vi "demo.vi"() -> ()   [LabVIEW 2009]
uses:
  <vilib>/Utility/miscctls.llb/LVPositionTypeDef.ctl
panel:
  in  "exit":bool
  in  "type":i8(ring) items=["甲", "乙", "丙", "丁"]
  in  "listbox":i32(listbox)
  # "演示列表框"
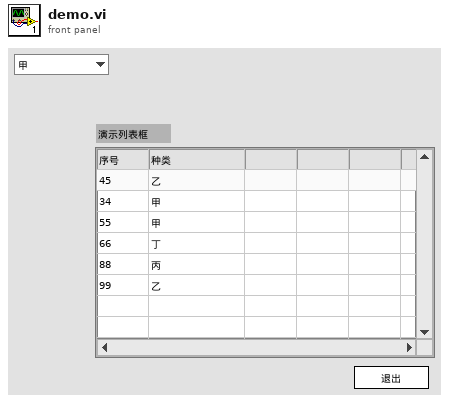
[diagram p1: front panel]
types:
  T1 = typedef "LVPositionTypeDef.ctl" = cluster{"Left":i32, "Top":i32}
  T2 = typedef "LVRowAndColumnTypeDef.ctl" = cluster{"Row":i32, "Column":i32}
  T3 = typedef "LVPoint32TypeDef.ctl" = cluster{"Horizontal":i32, "Vertical":i32}
  T4 = typedef "LVBoundsTypeDef.ctl" = cluster{"Width":u32, "Height":u32}
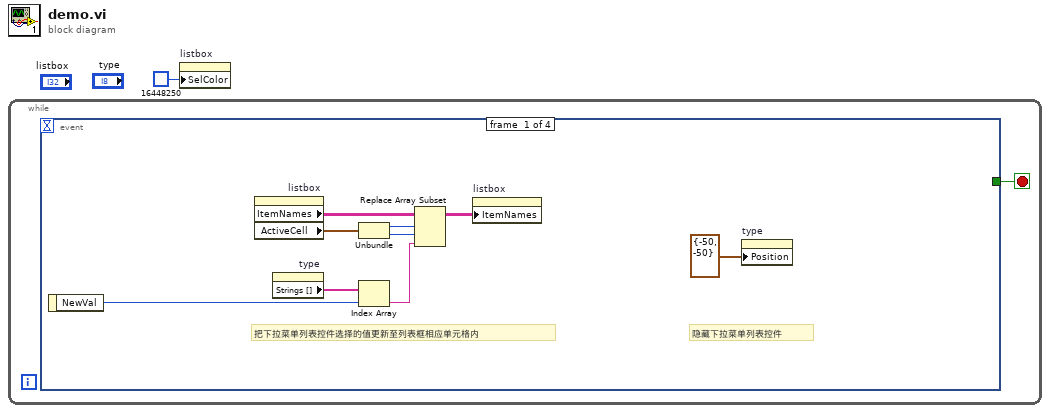
[diagram p0: block diagram]
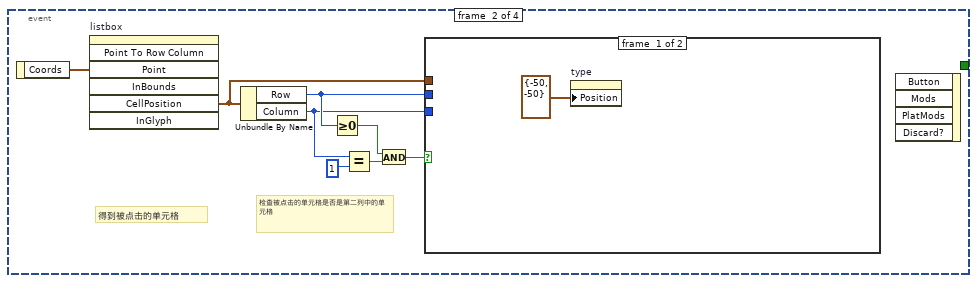
[diagram p2: hidden frame]
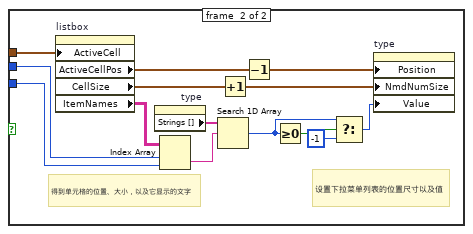
[diagram p3: hidden frame]
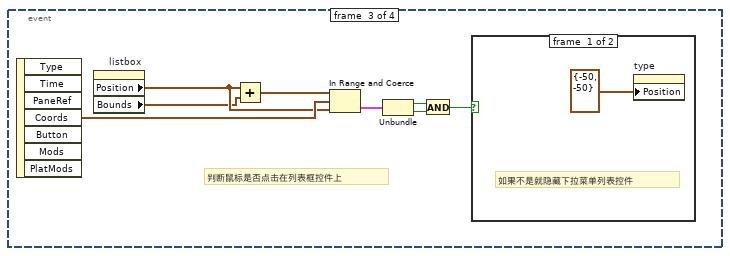
[diagram p4: hidden frame]
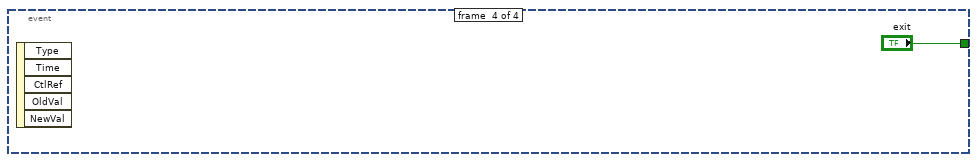
[diagram p6: hidden frame]
diagram:
  n1 = while {
    stop <- w2 stop-if-true
    n2 = event shown="[1] \"listbox\": Mouse Down?" {
      selector: _ -> [_ _ _ _]
      dyn-events: _ -> [_ _ _ _]
      timeout: _ -> [_ _ _ _]
      tunnel: [_ _ _ "exit"] -> w2
      event #0 {
        # "隐藏下拉菜单列表控件"
        # "把下拉菜单列表控件选择的值更新至列表框相应单元格内"
        n3 = event-data() -> ("NewVal"=w10:i8)  [unwired: 1 in]
        n4 = property on="listbox" class="MCListbox (strict)"() -> ("ItemNames"=w9:string[][], "ActiveCell"=w8:T2)  [unwired: 2 in, 2 out]
        n5 = property on="type" class="Ring (strict)"() -> ("Strings []"=w11:string[])  [unwired: 2 in, 2 out]
        n6 = Unbundle(w8) -> ("Row"=w7:i32, "Column"=w6:i32)
        n7 = Index Array(array=w11, index=w10) -> (element=w4:string)
        n8 = Replace Array Subset(array=w9, new element=w4, index (row)=w7, index (col)=w6) -> (w5:string[][])
        n9 = property on="listbox" class="MCListbox (strict)"("ItemNames"=w5) -> ()  [unwired: 2 in, 2 out]
        n10 = property on="type" class="Ring (strict)"("Position"=T1 {"Left"=-50, "Top"=-50}) -> ()  [unwired: 2 in, 2 out]
      }
      event #1 {
        # "检查被点击的单元格是否是第二列中的单元格"
        # "得到被点击的单元格"
        n11 = event-data() -> ("Coords"=w19:T3)  [unwired: 1 in]
        n12 = invoke on="listbox" class="MCListbox (strict)" method="Point To Row Column"("Point"=w19) -> ("CellPosition"=w12:T2)  [unwired: 6 in, 6 out]
        n13 = Unbundle By Name(w12) -> ("Row"=w14:i32, "Column"=w13:i32)
        n14 = Greater Or Equal To 0?(x=w14) -> (x >= 0?=w17:bool)
        n15 = Equal?(x=w13, y=1) -> (x = y?=w16:bool)
        n16 = And(x=w17, y=w16) -> (x .and. y?=w15:bool)
        n17 = case shown="True" w15 {
          tunnel: w14 -> [_ w33]
          tunnel: w13 -> [_ w32]
          tunnel: w12 -> [_ w31]
          frame #0 {
            n18 = property on="type" class="Ring (strict)"("Position"=T1 {"Left"=-50, "Top"=-50}) -> ()  [unwired: 2 in, 2 out]
          }
          frame #1 {
            # "设置下拉菜单列表的位置尺寸以及值"
            # "得到单元格的位置、大小，以及它显示的文字"
            n19 = property on="listbox" class="MCListbox (strict)"("ActiveCell"=w31) -> ("ActiveCellPos"=w27:T1, "CellSize"=w28:T4, "ItemNames"=w34:string[][])  [unwired: 2 in, 2 out]
            n20 = property on="type" class="Ring (strict)"() -> ("Strings []"=w29:string[])  [unwired: 2 in, 2 out]
            n21 = Index Array(array=w34, index (row)=w33, index (col)=w32) -> (element=w30:string)
            n22 = Search 1D Array(1D array=w29, element=w30) -> (index of element=w24:i32)  [unwired: 1 in]
            n23 = Increment(x=w28) -> (x+1=w21:T4)
            n24 = Decrement(x=w27) -> (x-1=w26:T1)
            n25 = Greater Or Equal To 0?(x=w24) -> (x >= 0?=w25:bool)
            n26 = Select(t=w24, s=w25, f=-1) -> (s? t:f=w22:i32)
            n27 = property on="type" class="Ring (strict)"("Position"=w26, "NmdNumSize"=w21, "Value"=w22) -> ()  [unwired: 2 in, 2 out]
          }
        }
        n28 = event-data() -> ()  [unwired: 5 in, 1 out]
      }
      event #2 {
        # "判断鼠标是否点击在列表框控件上"
        n29 = event-data() -> ("Coords"=w42:T3)  [unwired: 1 in, 6 out]
        n30 = property on="listbox" class="MCListbox (strict)"() -> ("Position"=w41:T1, "Bounds"=w40:T4)  [unwired: 2 in, 2 out]
        n31 = Add(x=w41, y=w40) -> (x+y=w39:T4)
        n32 = In Range and Coerce(upper limit=w39, x=w42, lower limit=w41) -> (In Range?=w38:cluster{"Width":bool, "Height":bool})  [unwired: 1 out]
        n33 = Unbundle(w38) -> ("Width"=w37:bool, "Height"=w36:bool)
        n34 = And(x=w37, y=w36) -> (x .and. y?=w35:bool)
        n35 = case shown="False" w35 {
          frame #0 {
            # "如果不是就隐藏下拉菜单列表控件"
            n36 = property on="type" class="Ring (strict)"("Position"=T1 {"Left"=-50, "Top"=-50}) -> ()  [unwired: 2 in, 2 out]
          }
          frame #1 {
          }
        }
      }
      event #3 {
        n37 = event-data() -> ()  [unwired: 1 in, 5 out]
      }
    }
  }
  n38 = property on="listbox" class="MCListbox (strict)"("SelColor"=u32 16448250) -> ()  [unwired: 2 in, 2 out]
